vi "XML-to-Array.vi"() -> (0 "Weights (4x9)":dbl[][](array[numeric]), 1 "Weights (4x4x15x8)":dbl[][][][](array[numeric]), 2 "Weights (4x4x1000x15)":dbl[][][][](array[numeric]), 3 "Weights (1000x2001)":dbl[][](array[numeric]))   [LabVIEW 2020]
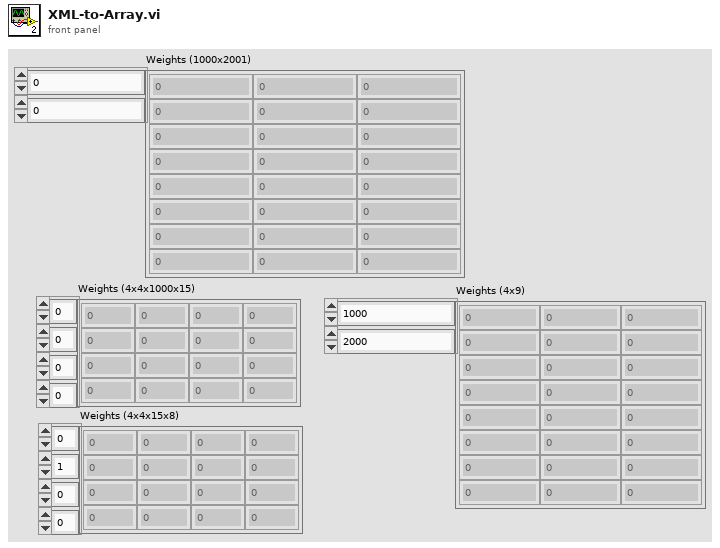
[diagram p1: front panel]
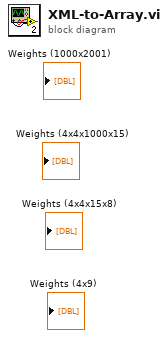
[diagram p0: block diagram]
diagram:
